vi "Inverse f Settings Check.vi"(6 "fs":dbl=1.0 format="%.2f", 7 "exponent":dbl=1.0 format="%.2g", 9 "order":i32=5, 10 "higher cutoff freq":dbl=0.5, 11 "lower cutoff freq":dbl=0.1) -> (2 "error index":i32, 3 "error code":i32)   [LabVIEW 2010, in "NI_AALBase.lvlib"]
doc: "Checks to make sure that each inverse f filter design parameter is within a valid range."
uses:
  NI_AALBase.lvlib
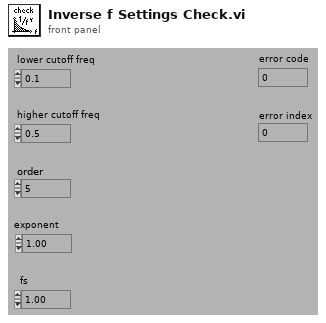
[diagram p1: front panel]
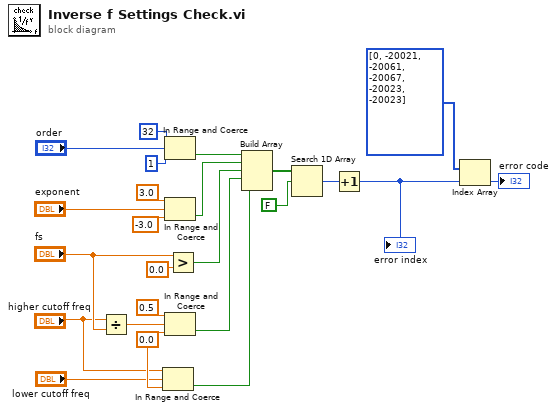
[diagram p0: block diagram]
diagram:
  w7 = 0.0
  n1 = Divide(x="higher cutoff freq", y="fs") -> (x/y=w6:dbl)
  n2 = In Range and Coerce(upper limit="higher cutoff freq", x="lower cutoff freq", lower limit=w7) -> (In Range?=w5:bool)  [unwired: 1 out]
  n3 = In Range and Coerce(upper limit=32, x="order", lower limit=1) -> (In Range?=w17:bool)  [unwired: 1 out]
  n4 = In Range and Coerce(upper limit=3.0, x="exponent", lower limit=-3.0) -> (In Range?=w16:bool)  [unwired: 1 out]
  n5 = In Range and Coerce(upper limit=0.5, x=w6, lower limit=w7) -> (In Range?=w10:bool)  [unwired: 1 out]
  n6 = Greater?(x="fs", y=0.0) -> (0:w11:bool)
  n7 = Build Array(w17, w16, w11, w10, w5) -> (w15:bool[])
  n8 = Search 1D Array(1D array=w15, element=FALSE) -> (index of element=w12:i32)  [unwired: 1 in]
  n9 = Increment(x=w12) -> (x+1=w8:i32)
  "error index" <- w8
  n10 = Index Array(array=i32[] [0, -20021, -20061, -20067, -20023, -20023], index=w8) -> (element=→"error code":i32)
